vi "Add Parameter Channel.vi"(8 "error in":errorcluster, 9 "channel definition":T2, 10 "name":string, 11 "section":T1 format="%.0x") -> (0 "error out":errorcluster, 2 "channel":T1 format="%.0x", 3 "section out":T1 format="%.0x")   [LabVIEW 2020, in "AIM MIL-STD-1553 Scripting.lvlib"]
doc: "Adds a channel to the specified <b>section</b> of the system definition."
uses:
  AIM MIL-STD-1553 Scripting.lvlib
  <vilib>/NI VeriStand/Custom Device API/Custom Device API.lvlib
  Constants.vi
  <vilib>/NI VeriStand/Custom Device API/Custom Device Item Ref.ctl
  <vilib>/NI VeriStand/Custom Device API/Custom Device Channel Type.ctl
  <vilib>/NI VeriStand/Custom Device API/Custom Device Channel.ctl
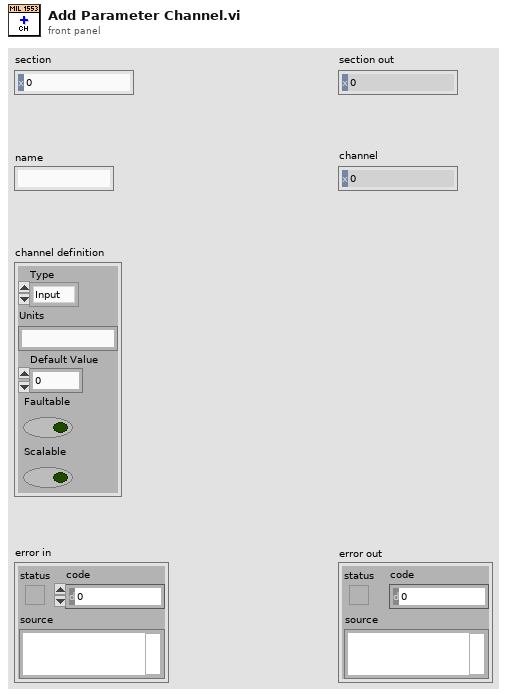
[diagram p1: front panel]
types:
  T1 = typedef "Custom Device API.lvlib/Custom Device Item Ref.ctl" = u64
  T2 = typedef "Custom Device API.lvlib/Custom Device Channel.ctl" = cluster{"Type":T3, "Units":string, "Default Value":dbl, "Faultable":bool, "Scalable":bool}
  T3 = typedef "Custom Device API.lvlib/Custom Device Channel Type.ctl" = enum16{"Input", "Output"}
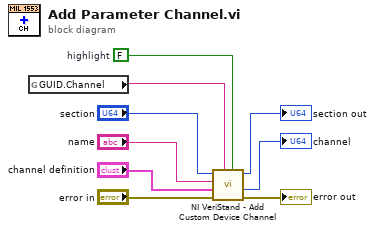
[diagram p0: block diagram]
diagram:
  w3 = FALSE  # highlight
  n1 = global read "Constants.vi" "GUID.Channel"() -> (w2:string)
  n2 = call <vilib>:"NI VeriStand - Add Custom Device Channel.vi"("Highlight? (F)"=w3, "GUID (Default Channel)"=w2, "error in (no error)"="error in", "Channel"="channel definition", "Channel Name"="name", "Parent Ref in"="section") -> ("error out"=→"error out":errorcluster, "Channel Ref"=→"channel":T1, "Parent Ref out"=→"section out":T1)  [unwired: 2 in, 1 out]
